vi "Barcode scanner lisen MIC.vi"(8 "error out 3":errorcluster, 10 "port":u16=1000, 11 "service name":string="192.168.1.20") -> (0 "error out 2":errorcluster, 2 "Exit":bool, 3 "data out":string)   [LabVIEW 2015]
uses:
  Galobal variable_TI.vi
panel:
  out "Numeric":i32
  out "error out":errorcluster
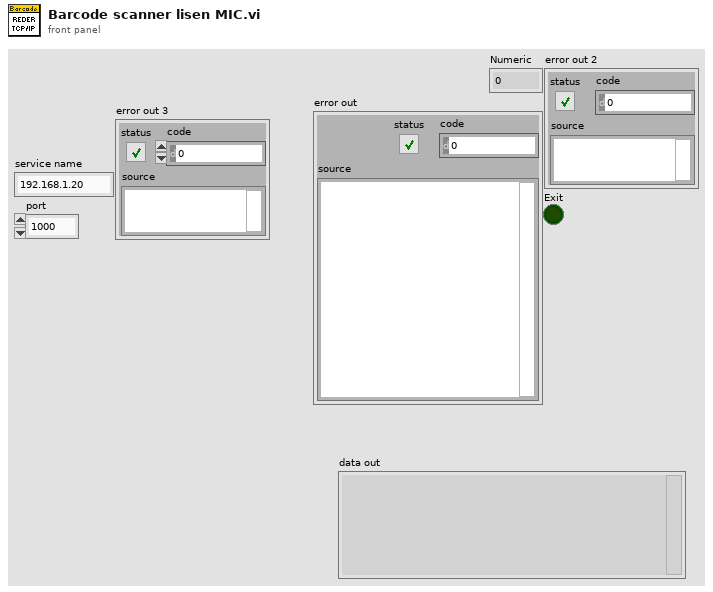
[diagram p1: front panel]
types:
  T1 = enum16{"Standard", "Buffered", "CRLF", "Immediate"}
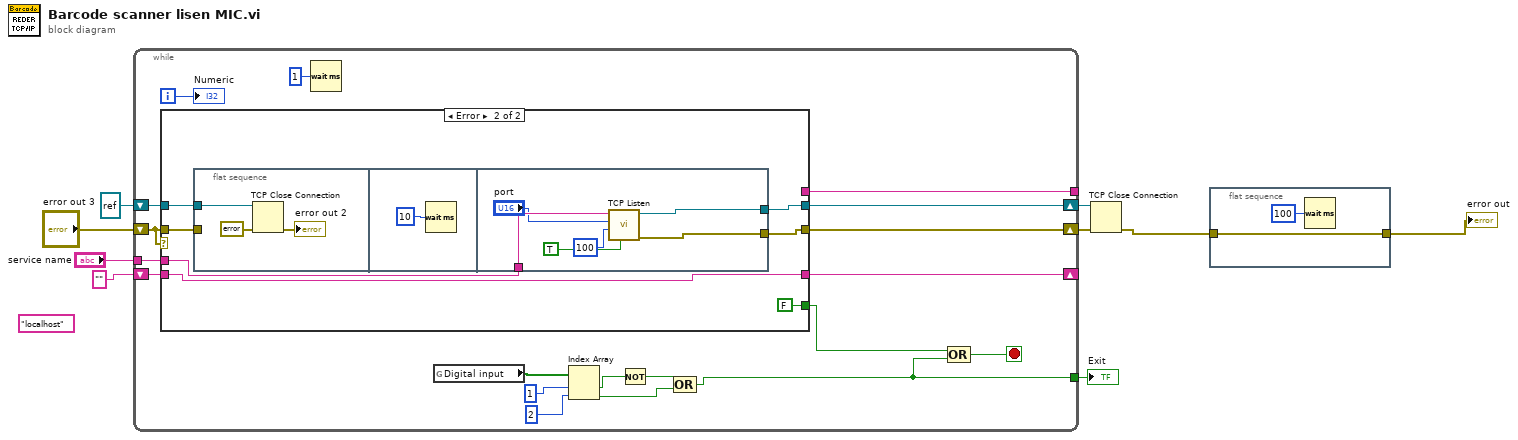
[diagram p0: block diagram]
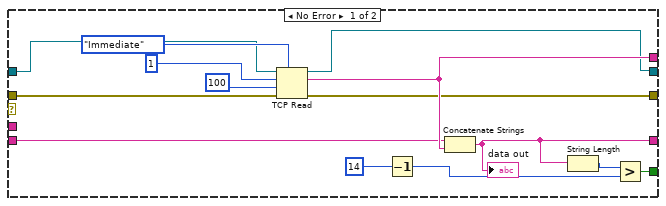
[diagram p2: hidden frame]
diagram:
  (unwired) "localhost" ("service name")
  n1 = while {
    tunnel: [w26] -> _
    shift-right: [w28] -> w9
    shift-left: refnum<k5> refnum ("connection ID") -> [w25]
    shift-right: [w27] -> w8
    shift-left: "error out 3" -> [w24]
    tunnel: "service name" -> [w23]
    shift-right: [w22] -> _
    shift-left: "" -> [w21]
    tunnel: [w10] -> w3
    i -> [w20]
    stop <- w17 stop-if-true
    n2 = case shown="Error" w24 {
      tunnel: [w37 w45] -> w28
      tunnel: [w36 w44] -> w27
      tunnel: [w39 _] -> w26
      tunnel: w25 -> [w41 w49]
      tunnel: w24 -> [w40 w48]
      tunnel: w23 -> [_ w47]
      tunnel: [w34 w46] -> w22
      tunnel: w21 -> [w38 w46]
      tunnel: [w32 FALSE] -> w18
      frame No Error {
        n3 = TCP Read(connection ID=w41, bytes to read=1, error in (no error)=w40, 7:T1."Immediate" ("mode (standard)"), 9:100 ("timeout ms (25000)")) -> (connection ID out=w37:refnum<k5>, data out=w39:string, error out=w36:errorcluster)
        n4 = Decrement(x=14) -> (x-1=w30:i32)
        n5 = Concatenate Strings(w38, w39) -> (w34:string)
        "data out" <- w34
        n6 = String Length(string=w34) -> (length=w33:i32)
        n7 = Greater?(x=w33, y=w30) -> (0:w32:bool)
      }
      frame Error {
        n8 = flat-sequence {
          tunnel: w49 -> [w52]
          tunnel: w48 -> [_]
          tunnel: w47 -> [w58]
          tunnel: [w57] -> w45
          tunnel: [w56] -> w44
          frame #0 {
            n9 = TCP Close Connection(connection ID=w52, error in (no error)=errorcluster {"status"=FALSE, "code"=0, "source"=""}) -> (error out=→"error out 2":errorcluster)  [unwired: 1 in, 1 out]
          }
          frame #1 {
            n10 = Wait (ms)(milliseconds to wait=u32 10) -> ()  [unwired: 1 out]
          }
          frame #2 {
            n11 = call <vilib>:"TCP Listen.vi"("resolve remote address (T)"=TRUE, "timeout ms (wait forever: -1)"=100, "port"="port", "service name"=w58) -> ("error out"=w56:errorcluster, "connection ID"=w57:refnum<k5>)  [unwired: 3 in, 3 out]
          }
        }
      }
    }
    n12 = Wait (ms)(milliseconds to wait=u32 1) -> ()  [unwired: 1 out]
    n13 = global read "Galobal variable_TI.vi" "Digital input"() -> (w16:bool[])
    n14 = Index Array(array=w16, index #1=1 ("index"), index #2=2 ("index")) -> (element #1=w13:bool, element #2=w11:bool)
    n15 = Not(x=w13) -> (.not. x?=w12:bool)
    n16 = Compound Arithmetic op=OR(w12, w11) -> (w10:bool)
    n17 = Compound Arithmetic op=OR(w18, w10) -> (w17:bool)
    "Numeric" <- w20
  }
  "Exit" <- w3
  n18 = TCP Close Connection(connection ID=w9, error in (no error)=w8) -> (error out=w2:errorcluster)  [unwired: 1 in, 1 out]
  n19 = flat-sequence {
    tunnel: w2 -> [w61]
    tunnel: [w61] -> w1
    frame #0 {
      n20 = Wait (ms)(milliseconds to wait=u32 100) -> ()  [unwired: 1 out]
    }
  }
  "error out" <- w1
